vi "Homogeneity_C_V_M.vi"(8 "error in (no error)":errorcluster caption="entrée d'erreur (pas d'erreur)", 9 "labels_pred":string[][](array[string]), 10 "labels_true":string[][](array[string]), 11 "homogeneity_completeness_v_measure":cluster{"beta":dbl, "Returns":string}={"beta"=1.0, "Returns"="homogeneity"}) -> (0 "error out":errorcluster caption="sortie d'erreur", 3 "Score":string)   [LabVIEW 2020]
doc: "Compute the homogeneity and completeness and V-Measure scores at once.\n\nThose metrics are based on normalized conditional entropy measures of the clustering labeling to evaluate given the knowledge of a Ground Truth class labels of the same samples.\n\nA clustering result satisfies homogeneity if all of its clusters contain only data points which are members of a single class.\n\nA clustering result satisfies completeness if all the data points that are members of a given class are elements of the same cluster.\n\nBoth scores have positive values between 0.0 and 1.0, larger values being desirable.\n\nThose 3 metrics are independent of the absolute values of the labels: a permutation of the class or cluster label values won’t change the score values in any way.\n\nV-Measure is furthermore symmetric: swapping labels_true and label_pred will give the same score. This does not hold for homogeneity and completeness. V-Measure is identical to normalized_mutual_info_score with the arithmetic averaging method.\n\n\n\nParameters : \n\n- labels_true : int array, shape = [n_samples]\nground truth class labels to be used as a reference\n\n- labels_pred : array-like of shape (n_samples,)\ncluster labels to evaluate\n\n- beta : float\nRatio of weight attributed to homogeneity vs completeness. If beta is greater than 1, completeness is weighted more strongly in the calculation. If beta is less than 1, homogeneity is weighted more strongly.\n\nReturns : \n\n- homogeneity : float\nscore between 0.0 and 1.0. 1.0 stands for perfectly homogeneous labeling\n\n- completeness : float\nscore between 0.0 and 1.0. 1.0 stands for perfectly complete labeling\n\n- v_measure : float\nharmonic mean of the first two"
uses:
  Homogeneity_C_V_M.lvclass
panel:
  out "Homogeneity_C_V_M.lvclass":refnum<class "Homogeneity_C_V_M.lvclass">
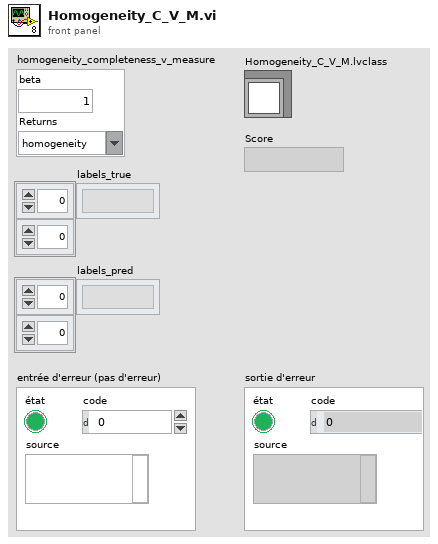
[diagram p1: front panel]
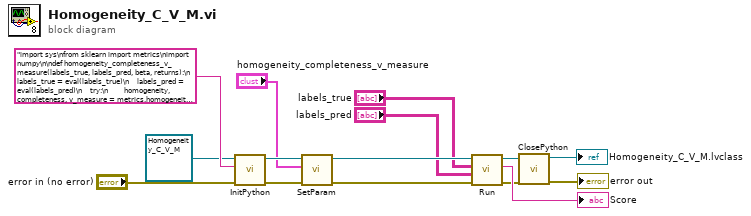
[diagram p0: block diagram]
diagram:
  n1 = call-dynamic "InitPython.vi"("error in (no error)"="error in (no error)", "Python Instruction"="import sys\nfrom sklearn import metrics\nimport numpy\n\ndef homogeneity_completeness_v_measure(labels_true, labels_pred, beta, returns):\n    labels_true = eval(labels_true)\n    labels_pred = eval(labels_pred)\n    try:\n        homogeneity, completeness, v_measure = metrics.homogeneity_completeness_v_measure(labels_true, labels_pred, beta)\n        if returns == 'homogeneity':\n            homogeneity_completeness_v_measure = homogeneity.tolist()\n            return str(homogeneity_completeness_v_measure)\n        elif returns == 'completeness':\n            homogeneity_completeness_v_measure = completeness.tolist()\n            return str(homogeneity_completeness_v_measure)\n        else:\n            homogeneity_completeness_v_measure = v_measure.tolist()\n            return str(homogeneity_completeness_v_measure)\n    except:\n        erreur = sys.exc_info()\n        typerr = u\"%s\" % (erreur[0])\n        typerr = typerr[typerr.find(\"'\")+1:typerr.rfind(\"'\")]\n        msgerr = u\"%s\" % (erreur[1])\n        message = str('/!\\\\ {0} : {1}'. format(typerr,msgerr))\n        return message", "Scikit-learn en entrée"=refnum<class "Homogeneity_C_V_M.lvclass"> refnum ("Homogeneity_C_V_M.lvclass")) -> ("error out"=w9:errorcluster, "Scikit-learn en sortie"=w11:refnum<class "Homogeneity_C_V_M.lvclass">)  [unwired: 7 in]
  n2 = call-dynamic "SetParam.vi"("error in (no error)"=w9, "homogeneity_completeness_v_measure"="homogeneity_completeness_v_measure", "Homogeneity_C_V_M.lvclass"=w11) -> ("error out"=w7:errorcluster, "Homogeneity_C_V_M.lvclass"=w8:refnum<class "Homogeneity_C_V_M.lvclass">)  [unwired: 7 in]
  n3 = call-dynamic "Run.vi"("error in (no error)"=w7, "labels_pred"="labels_pred", "labels_true"="labels_true", "Homogeneity_C_V_M.lvclass"=w8) -> ("error out"=w5:errorcluster, "String Data"=→"Score":string, "Homogeneity_C_V_M.lvclass"=w4:refnum<class "Homogeneity_C_V_M.lvclass">)  [unwired: 5 in]
  n4 = call-dynamic "ClosePython.vi"("error in (no error)"=w5, "Scikit-learn en entrée"=w4) -> ("error out"=→"error out":errorcluster, "Scikit-learn en sortie"=→"Homogeneity_C_V_M.lvclass":refnum<class "Homogeneity_C_V_M.lvclass">)  [unwired: 8 in]
